vi "stage-controller.vi"() -> ()   [LabVIEW 2014]
uses:
  Stage SubVIs/ctts/move stage.ctl
  stage-controller-globals.vi
  Library Files - Andor and MadCity/Madlib/Madlib.lvlib
panel:
  in  "Current Z 2":ext(slide)=5.551115123125783e-17 scale=-1.0..1.0 scale format="%_1f"
  out "Current (X,Y)":cluster{ext[], ext[]}[](graph)=[{[101.064], [100.915]}, {[101.064, 151.59599999999998], [100.915, 100.915]}, {[101.064, 151.59599999999998], [50.457499999999996, 50.457499999999996]}]
  in  "Field Number":u32(slide)=1 min=1 max=16 step=1 scale=1.0..16.0
  in  "Field Size":enum16{"0", "1", "4", "9", "16"}(ring)=enum."16"
  in  "x-":bool
  in  "y+":bool
  in  "y-":bool
  in  "x+":bool
  out "Current Z (um)":ext=101.117
  out "Current X (um)":ext=101.064
  out "Current Y (um)":ext=100.915
  in  "Current Z":dbl(slide)=101.5 min=0.0 step=0.5 scale=0.0..202.234 scale format="%#_4g"
  out "At limit 3":bool
  out "At limit 2":bool
  out "At limit":bool
  in  "x,y step (um)":ext=10.0 format="%_5g"
  in  "z step (um)":ext(slide)=0.1 scale=0.05..2.0 scale format="%#_2g"
  in  "z-":bool
  in  "z+":bool
  in  "Reset stage to center\n         (x, y, and z)":bool
  in  "STOP":bool
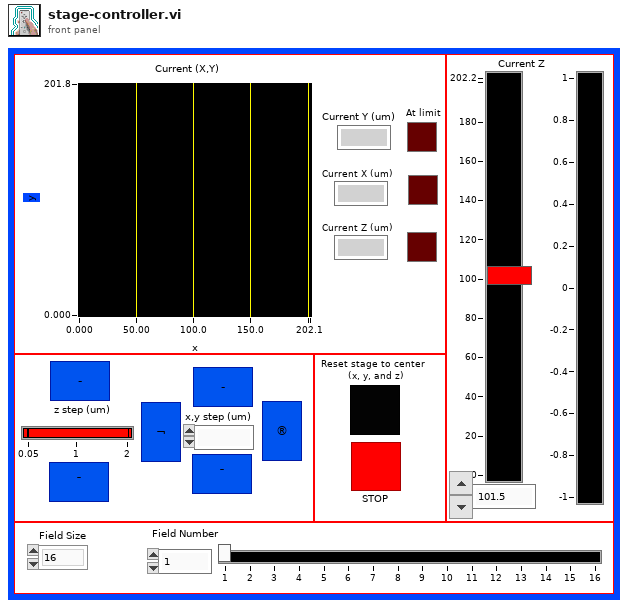
[diagram p1: front panel]
types:
  T1 = cluster{"X Command":dbl, "Y Command":dbl, "Z Command":dbl, "X Position":dbl, "Y Position":dbl, "Z Position":dbl, "X Calibration":dbl, "Y Calibration":dbl, "Z Calibration":dbl}
  T2 = typedef "move stage.ctl" = cluster{"dx (um) (0 -> ignore)":ext, "dy (um) (0 -> ignore)":ext, "dz (um) (0 -> ignore)":ext, "Re-center x,y":bool, "Re-center z":bool, "x (um) (-1 -> ignore)":dbl, "y (um) (-1 -> ignore)":dbl, "z (um) (-1 -> ignore)":dbl, "Move to Next Field":bool}
  T3 = typedef "small z increment.ctl" = dbl
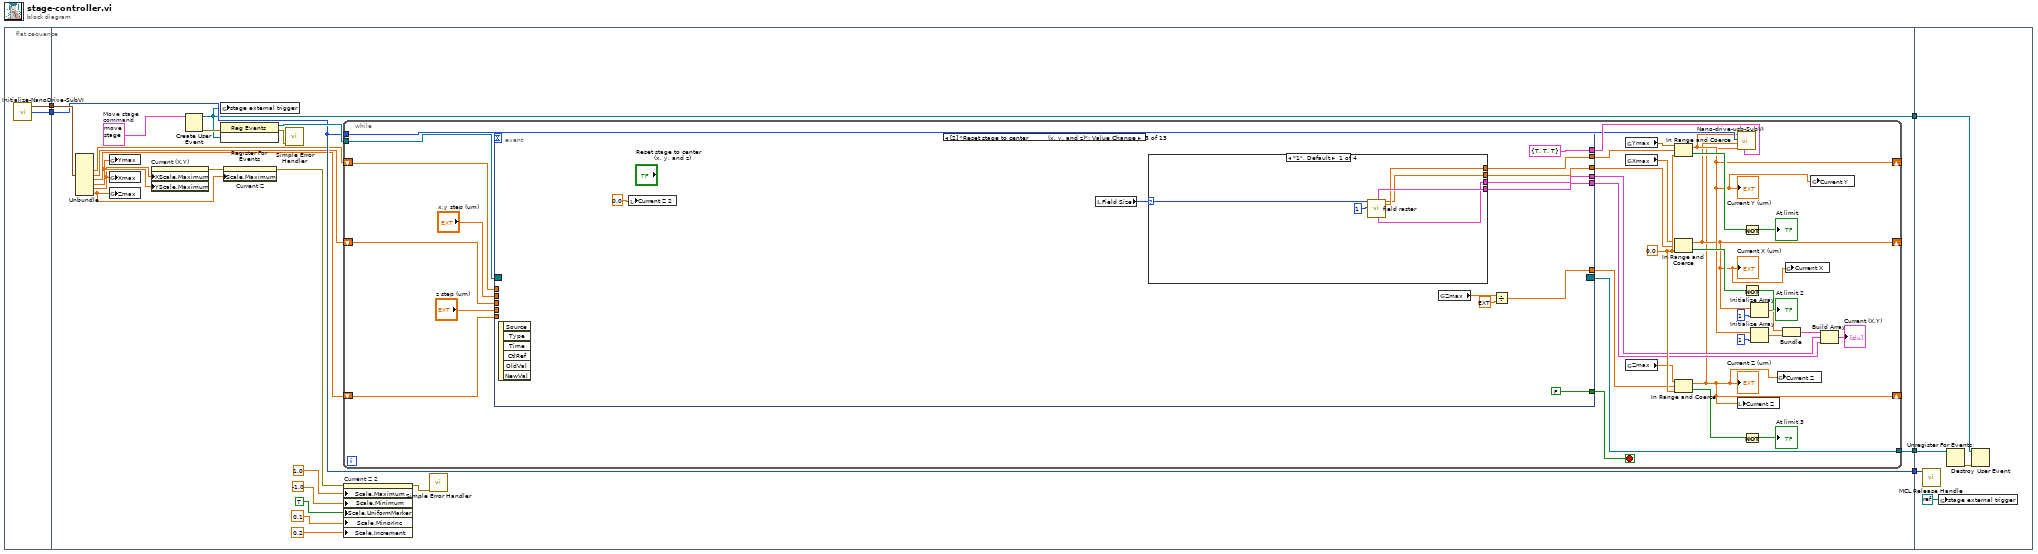
[diagram p0: block diagram]
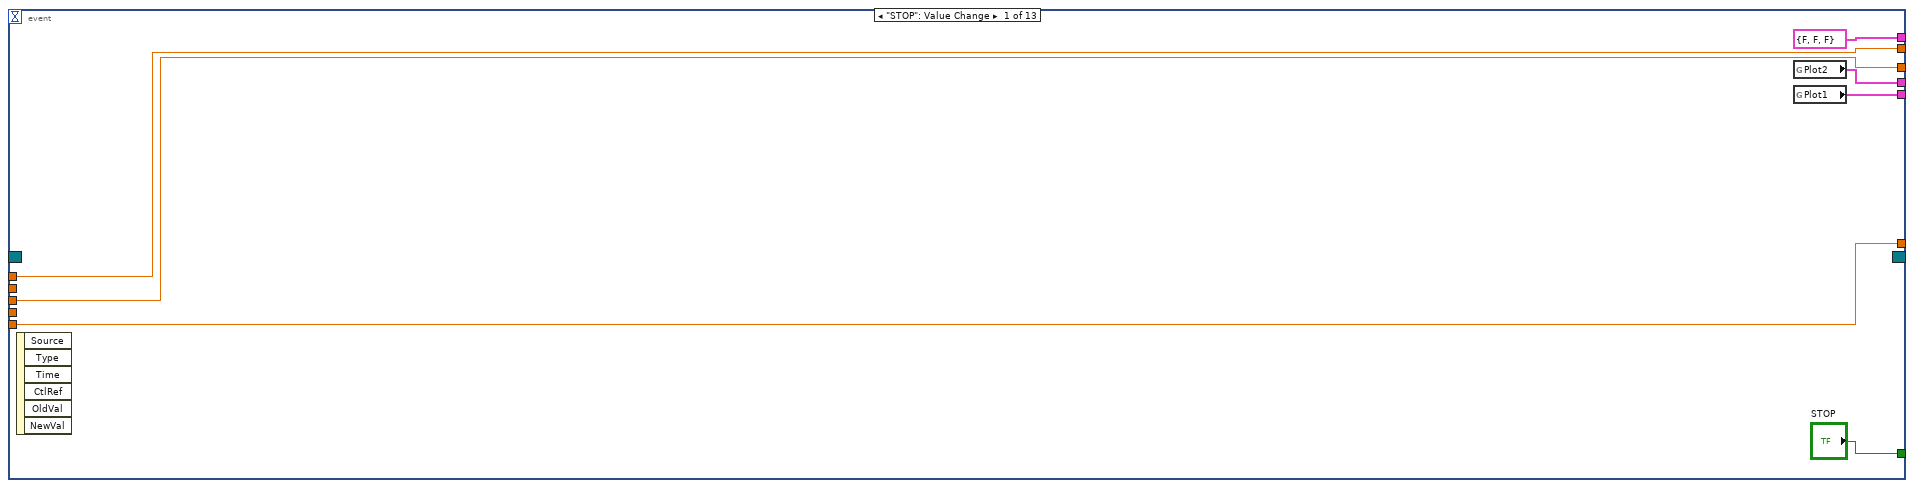
[diagram p2: hidden frame]
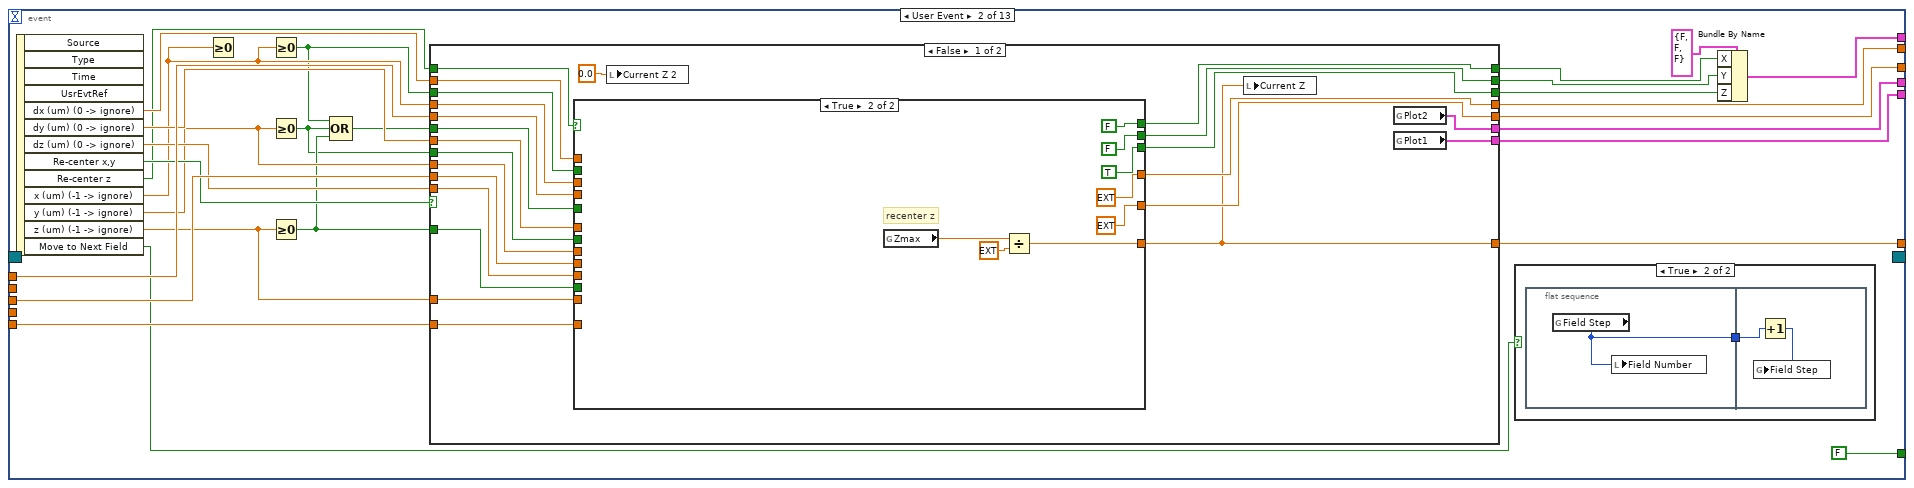
[diagram p3: hidden frame]
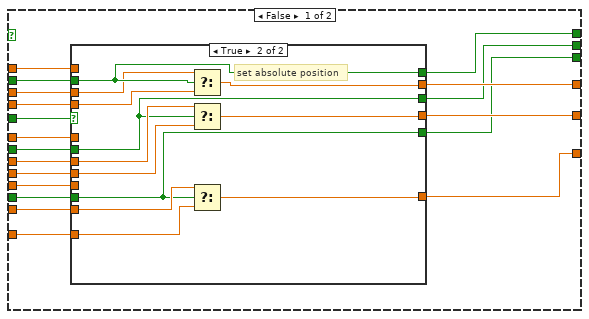
[diagram p5: hidden frame]
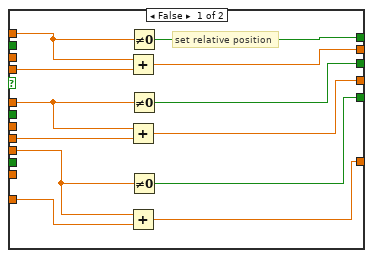
[diagram p6: hidden frame]
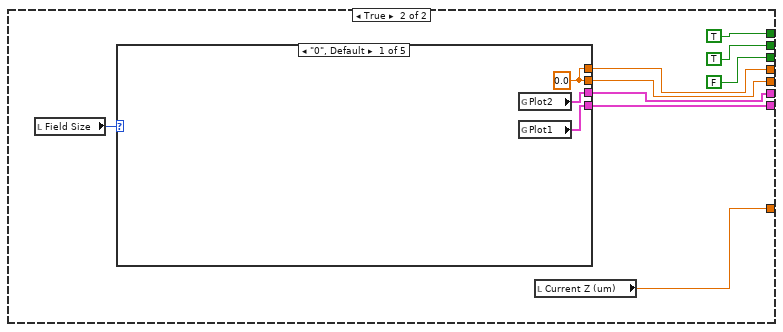
[diagram p7: hidden frame]
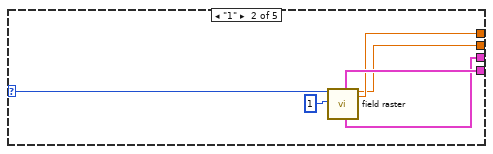
[diagram p8: hidden frame]
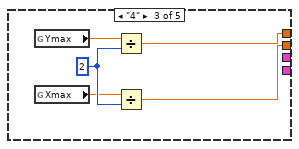
[diagram p9: hidden frame]
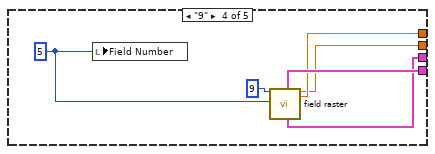
[diagram p10: hidden frame]
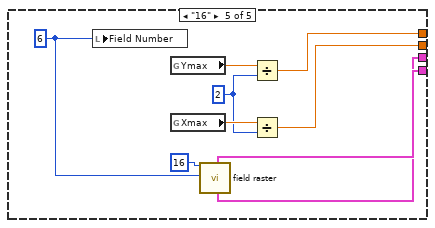
[diagram p11: hidden frame]
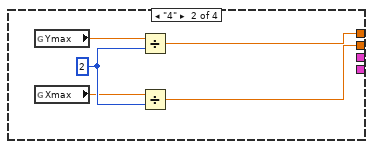
[diagram p12: hidden frame]
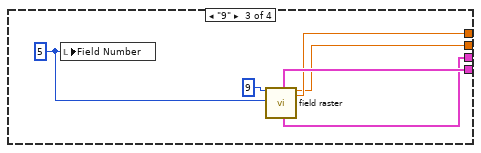
[diagram p13: hidden frame]
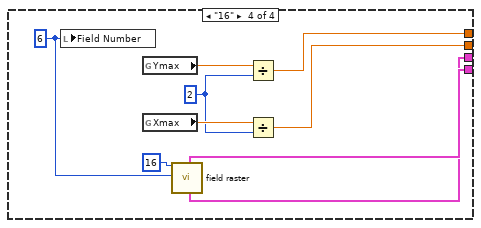
[diagram p14: hidden frame]
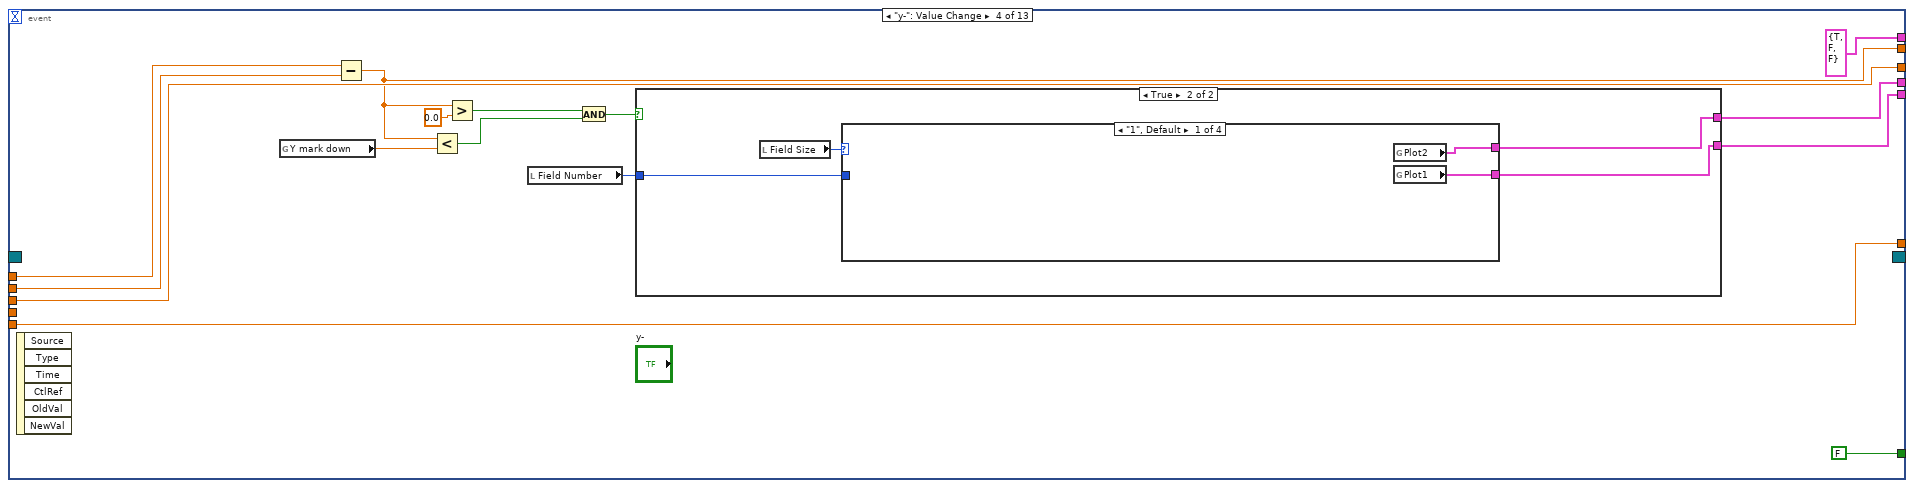
[diagram p15: hidden frame]
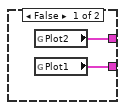
[diagram p16: hidden frame]
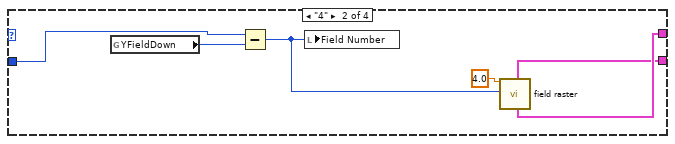
[diagram p17: hidden frame]
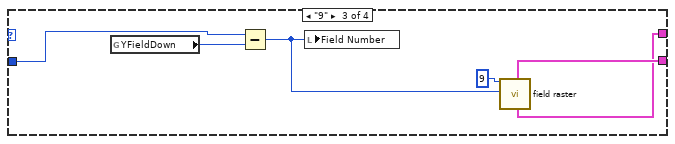
[diagram p18: hidden frame]
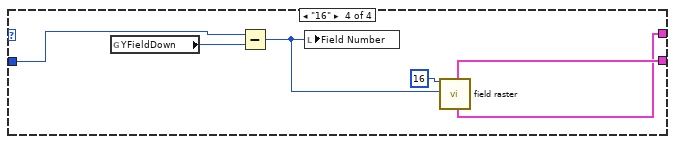
[diagram p19: hidden frame]
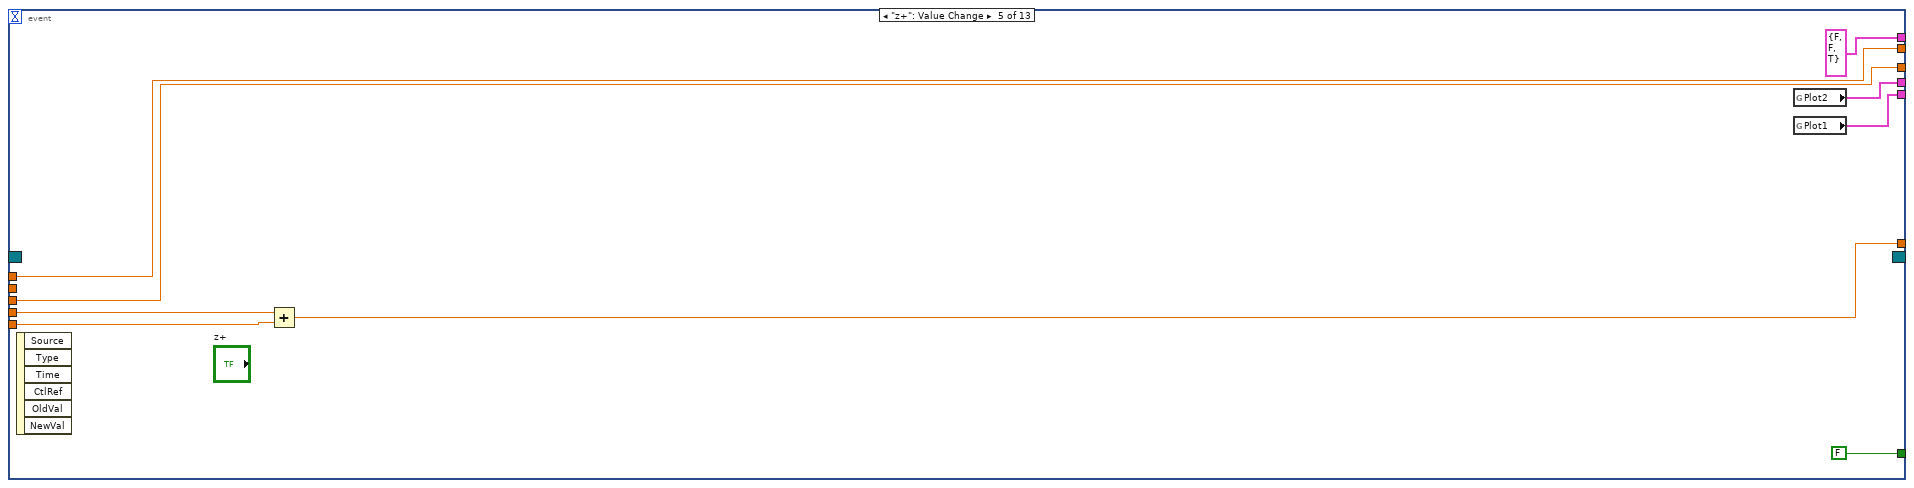
[diagram p20: hidden frame]
diagram:
  n1 = flat-sequence {
    tunnel: [w7] -> w5
    tunnel: [w6] -> w2
    tunnel: w5 -> [w29]
    tunnel: [w24] -> w4
    tunnel: [w8] -> w3
    tunnel: w2 -> [w23]
    tunnel: [w23] -> w1
    tunnel: w4 -> [w498]
    tunnel: w3 -> [w497]
    tunnel: w1 -> [w496]
    frame #0 {
      n2 = call "Initialize-NanoDrive-SubVI.vi"() -> ("Output Pos Info"=w7:T1, "Handle"=w6:i32)  [unwired: 1 in, 1 out]
    }
    frame #1 {
      w28 = T2 {"dx (um) (0 -> ignore)"=0.0, "dy (um) (0 -> ignore)"=0.0, "dz (um) (0 -> ignore)"=0.0, "Re-center x,y"=FALSE, "Re-center z"=FALSE, "x (um) (-1 -> ignore)"=-1.0, "y (um) (-1 -> ignore)"=-1.0, "z (um) (-1 -> ignore)"=-1.0, "Move to Next Field"=FALSE}  # Move stage command
      n3 = Unbundle(w29) -> ("X Position"=w22:dbl, "Y Position"=w21:dbl, "Z Position"=w20:dbl, "X Calibration"=w18:dbl, "Y Calibration"=w17:dbl, "Z Calibration"=w16:dbl)  [unwired: 3 out]
      n4 = global write "stage-controller-globals.vi" "Ymax"(w18) -> ()
      n5 = global write "stage-controller-globals.vi" "Xmax"(w17) -> ()
      n6 = global write "stage-controller-globals.vi" "Zmax"(w16) -> ()
      n7 = property on="Current (X,Y)" class="XYGraph (strict)"("XScale.Maximum"=w17, "YScale.Maximum"=w18) -> (error out=w19:errorcluster)  [unwired: 2 in, 1 out]
      n8 = Create User Event(user event datatype=w28) -> (user event=w8:refnum<user-event>, error out=w26:errorcluster)  [unwired: 1 in]
      n9 = global write "stage-controller-globals.vi" "stage external trigger"(w8) -> ()
      n10 = register-events(error in=w26, w8) -> (reference out=w25:refnum<event-registration>, error out=w27:errorcluster)  [unwired: 1 in]
      n11 = property on="Current Z" class="Slide (strict)"(error in=w19, "Scale.Maximum"=w16) -> (error out=w15:errorcluster)  [unwired: 1 in, 1 out]
      n12 = call <vilib>:"Simple Error Handler.vi"("error in (no error)"=w27) -> ()  [unwired: 1 in, 8 out]
      n13 = while {
        tunnel: w25 -> [w61]
        tunnel: [w60] -> w24
        tunnel: w23 -> [w46]
        shift-right: [w32] -> _
        shift-left: w22 -> [w45]
        shift-right: [w31] -> _
        shift-left: w21 -> [w44]
        shift-right: [w30] -> _
        shift-left: w20 -> [w43]
        stop <- w62 stop-if-true
        w59 = 0.0
        n14 = event shown="[2] \"Reset stage to center          (x, y, and z)\": Value Change" {
          selector: w61 -> [_ _ _ _ _ _ _ _ _ _ _ _ _]
          dyn-events: [_ _ _ _ _ _ _ _ _ _ _ _ _] -> w60
          timeout: _ -> [_ _ _ _ _ _ _ _ _ _ _ _ _]
          tunnel: ["STOP" FALSE ("Stop") FALSE ("Stop") FALSE ("Stop") FALSE ("Stop") FALSE ("Stop") FALSE ("Stop") FALSE ("Stop") FALSE ("Stop") FALSE ("Stop") FALSE ("Stop") FALSE FALSE] -> w62
          tunnel: w45 -> [w69 w97 _ w261 w299 w306 w317 w336 w347 w392 w430 _ _]
          tunnel: w44 -> [w68 w96 _ w264 w294 w305 w316 w335 w351 w389 w434 _ _]
          tunnel: w43 -> [w67 w95 _ w263 w296 _ w314 w332 w352 w393 w433 _ _]
          tunnel: [w69 w92 w216 w252 w299 w306 w317 w336 w347 w392 w422 w465 w488] -> w58
          tunnel: [w68 w93 w217 w264 w294 w305 w316 w335 w340 w381 w434 w464 w487] -> w57
          tunnel: [w67 w94 w222 w263 w298 "Current Z" w313 w338 w352 w393 w433 w468 w483] -> w56
          tunnel: [cluster{"X":bool, "Y":bool, "Z":bool} {"X"=FALSE, "Y"=FALSE, "Z"=FALSE} ("Set this axis?") w85 cluster{"X":bool, "Y":bool, "Z":bool} {"X"=TRUE, "Y"=TRUE, "Z"=TRUE} ("Set this axis?") cluster{"X":bool, "Y":bool, "Z":bool} {"X"=TRUE, "Y"=FALSE, "Z"=FALSE} ("Set this axis?") cluster{"X":bool, "Y":bool, "Z":bool} {"X"=FALSE, "Y"=FALSE, "Z"=TRUE} ("Set this axis?") cluster{"X":bool, "Y":bool, "Z":bool} {"X"=FALSE, "Y"=FALSE, "Z"=TRUE} ("Set this axis?") cluster{"X":bool, "Y":bool, "Z":bool} {"X"=FALSE, "Y"=FALSE, "Z"=TRUE} ("Set this axis?") cluster{"X":bool, "Y":bool, "Z":bool} {"X"=FALSE, "Y"=FALSE, "Z"=TRUE} ("Set this axis?") cluster{"X":bool, "Y":bool, "Z":bool} {"X"=FALSE, "Y"=TRUE, "Z"=FALSE} ("Set this axis?") cluster{"X":bool, "Y":bool, "Z":bool} {"X"=FALSE, "Y"=TRUE, "Z"=FALSE} ("Set this axis?") cluster{"X":bool, "Y":bool, "Z":bool} {"X"=TRUE, "Y"=FALSE, "Z"=FALSE} ("Set this axis?") cluster{"X":bool, "Y":bool, "Z":bool} {"X"=FALSE, "Y"=FALSE, "Z"=FALSE} ("Set this axis?") cluster{"X":bool, "Y":bool, "Z":bool} {"X"=TRUE, "Y"=TRUE, "Z"=FALSE} ("Set this axis?")] -> w47
          tunnel: "x,y step (um)" -> [_ _ _ w260 _ _ _ _ w350 w390 w431 _ _]
          tunnel: "z step (um)" -> [_ _ _ _ w295 _ _ w333 _ _ _ _ _]
          tunnel: [w64 w72 w219 w257 w293 w302 w320 w331 w345 w386 w427 w463 w489] -> w38
          tunnel: [w65 w73 w220 w258 w292 w303 w319 w330 w346 w387 w428 w462 w490] -> w37
          event "STOP": Value Change {
            n15 = event-data() -> ()  [unwired: 7 out]
            n16 = global read "stage-controller-globals.vi" "Plot2"() -> (w64:cluster{dbl[], dbl[]})
            n17 = global read "stage-controller-globals.vi" "Plot1"() -> (w65:cluster{dbl[], dbl[]})
          }
          event User Event {
            n18 = event-data() -> ("dx (um) (0 -> ignore)"=w90:ext, "dy (um) (0 -> ignore)"=w89:ext, "dz (um) (0 -> ignore)"=w88:ext, "Re-center x,y"=w87:bool, "Re-center z"=w81:bool, "x (um) (-1 -> ignore)"=w77:dbl, "y (um) (-1 -> ignore)"=w78:dbl, "z (um) (-1 -> ignore)"=w79:dbl, "Move to Next Field"=w71:bool)  [unwired: 5 out]
            n19 = Greater Or Equal To 0?(x=w77) -> ()  [unwired: 1 out]
            n20 = Greater Or Equal To 0?(x=w77) -> (x >= 0?=w74:bool)
            n21 = Greater Or Equal To 0?(x=w78) -> (x >= 0?=w75:bool)
            n22 = Greater Or Equal To 0?(x=w79) -> (x >= 0?=w76:bool)
            n23 = Compound Arithmetic op=OR(w74, w75, w76) -> (w80:bool)
            n24 = case shown="False" w87 {
              tunnel: w97 -> [w124 _]
              tunnel: w96 -> [w123 _]
              tunnel: w95 -> [w122 _]
              tunnel: [w105 w177] -> w94
              tunnel: [w121 w179] -> w93
              tunnel: [w120 w178] -> w92
              tunnel: w90 -> [w119 _]
              tunnel: w89 -> [w118 _]
              tunnel: w88 -> [w117 _]
              tunnel: [w116 FALSE] -> w84
              tunnel: [w115 TRUE] -> w83
              tunnel: [w114 TRUE] -> w82
              tunnel: w81 -> [w113 _]
              tunnel: w80 -> [w112 _]
              tunnel: w79 -> [w111 _]
              tunnel: w78 -> [w110 _]
              tunnel: w77 -> [w109 _]
              tunnel: w76 -> [w108 _]
              tunnel: w75 -> [w107 _]
              tunnel: w74 -> [w106 _]
              tunnel: [w103 w181] -> w73
              tunnel: [w102 w180] -> w72
              frame False {
                n25 = case shown="True" w113 {
                  tunnel: w124 -> [w143 _]
                  tunnel: w123 -> [w142 _]
                  tunnel: w122 -> [w141 _]
                  tunnel: [w140 w174] -> w105
                  tunnel: [w139 ext 0.0] -> w121
                  tunnel: [w138 ext 0.0] -> w120
                  tunnel: w119 -> [w137 _]
                  tunnel: w118 -> [w136 _]
                  tunnel: w117 -> [w135 _]
                  tunnel: [w134 TRUE] -> w116
                  tunnel: [w133 FALSE] -> w115
                  tunnel: [w132 FALSE] -> w114
                  tunnel: w112 -> [w131 _]
                  tunnel: w111 -> [w130 _]
                  tunnel: w110 -> [w129 _]
                  tunnel: w109 -> [w128 _]
                  tunnel: w108 -> [w127 _]
                  tunnel: w107 -> [w126 _]
                  tunnel: w106 -> [w125 _]
                  frame False {
                    n26 = case shown="True" w131 {
                      tunnel: w143 -> [w155 w163]
                      tunnel: w142 -> [w154 w160]
                      tunnel: w141 -> [w153 w157]
                      tunnel: [w152 w159] -> w140
                      tunnel: [w151 w162] -> w139
                      tunnel: [w150 w166] -> w138
                      tunnel: w137 -> [w149 _]
                      tunnel: w136 -> [w148 _]
                      tunnel: w135 -> [w147 _]
                      tunnel: [w146 w156] -> w134
                      tunnel: [w145 w161] -> w133
                      tunnel: [w144 w165] -> w132
                      tunnel: w130 -> [_ w158]
                      tunnel: w129 -> [_ w167]
                      tunnel: w128 -> [_ w164]
                      tunnel: w127 -> [_ w156]
                      tunnel: w126 -> [_ w161]
                      tunnel: w125 -> [_ w165]
                      frame False {
                        # "set relative position"
                        n27 = Add(x=w149, y=w155) -> (x+y=w150:ext)
                        n28 = Add(x=w148, y=w154) -> (x+y=w151:ext)
                        n29 = Add(x=w147, y=w153) -> (x+y=w152:ext)
                        n30 = Not Equal To 0?(x=w149) -> (x != 0?=w144:bool)
                        n31 = Not Equal To 0?(x=w148) -> (x != 0?=w145:bool)
                        n32 = Not Equal To 0?(x=w147) -> (x != 0?=w146:bool)
                      }
                      frame True {
                        # "set absolute position"
                        n33 = Select(t=w164, s=w165, f=w163) -> (s? t:f=w166:ext)
                        n34 = Select(t=w167, s=w161, f=w160) -> (s? t:f=w162:ext)
                        n35 = Select(t=w158, s=w156, f=w157) -> (s? t:f=w159:ext)
                      }
                    }
                  }
                  frame True {
                    # "recenter z"
                    n36 = global read "stage-controller-globals.vi" "Zmax"() -> (w168:dbl)
                    n37 = Divide(x=w168, y=ext 2.0) -> (x/y=w174:ext)
                  }
                }
                n38 = local write "Current Z 2"(0.0) -> ()
                n39 = local write "Current Z"(w105) -> ()
                n40 = global read "stage-controller-globals.vi" "Plot2"() -> (w102:cluster{dbl[], dbl[]})
                n41 = global read "stage-controller-globals.vi" "Plot1"() -> (w103:cluster{dbl[], dbl[]})
              }
              frame True {
                n42 = local read "Field Size"() -> (w176:enum16{"0", "1", "4", "9", "16"})
                n43 = case shown="\"0\", Default" w176 {
                  selector: w176 -> [_ w191 _ _ _]
                  tunnel: [w186 w193 _ w202 w208] -> w181
                  tunnel: [w187 w192 _ w201 w207] -> w180
                  tunnel: [w185 w189 w198 w200 w211] -> w178
                  tunnel: [w185 w188 w197 w199 w210] -> w179
                  frame "0", Default {
                    w185 = 0.0
                    n44 = global read "stage-controller-globals.vi" "Plot2"() -> (w187:cluster{dbl[], dbl[]})
                    n45 = global read "stage-controller-globals.vi" "Plot1"() -> (w186:cluster{dbl[], dbl[]})
                  }
                  frame "1" {
                    n46 = call "field raster.vi"("field size"=w191, "field number"=1) -> ("Plot1"=w193:cluster{dbl[], dbl[]}, "Plot2"=w192:cluster{dbl[], dbl[]}, "current Y"=w188:dbl, "current X"=w189:dbl)  [unwired: 12 in, 2 out]
                  }
                  frame "4" {
                    w196 = 2
                    n47 = global read "stage-controller-globals.vi" "Ymax"() -> (w194:dbl)
                    n48 = global read "stage-controller-globals.vi" "Xmax"() -> (w195:dbl)
                    n49 = Divide(x=w194, y=w196) -> (x/y=w198:dbl)
                    n50 = Divide(x=w195, y=w196) -> (x/y=w197:dbl)
                  }
                  frame "9" {
                    w203 = 5
                    n51 = local write "Field Number"(w203) -> ()
                    n52 = call "field raster.vi"("field size"=9, "field number"=w203) -> ("Plot1"=w202:cluster{dbl[], dbl[]}, "Plot2"=w201:cluster{dbl[], dbl[]}, "current Y"=w199:dbl, "current X"=w200:dbl)  [unwired: 12 in, 2 out]
                  }
                  frame "16" {
                    w206 = 2
                    w205 = 6
                    n53 = local write "Field Number"(w205) -> ()
                    n54 = global read "stage-controller-globals.vi" "Ymax"() -> (w213:dbl)
                    n55 = global read "stage-controller-globals.vi" "Xmax"() -> (w212:dbl)
                    n56 = call "field raster.vi"("field size"=16, "field number"=w205) -> ("Plot1"=w208:cluster{dbl[], dbl[]}, "Plot2"=w207:cluster{dbl[], dbl[]})  [unwired: 12 in, 4 out]
                    n57 = Divide(x=w213, y=w206) -> (x/y=w211:dbl)
                    n58 = Divide(x=w212, y=w206) -> (x/y=w210:dbl)
                  }
                }
                n59 = local read "Current Z (um)"() -> (w177:ext)
              }
            }
            n60 = case shown="True" w71 {
              frame False {
              }
              frame True {
                n61 = flat-sequence {
                  tunnel: [w99] -> w98
                  tunnel: w98 -> [w101]
                  frame #0 {
                    n62 = global read "stage-controller-globals.vi" "Field Step"() -> (w99:u32)
                    n63 = local write "Field Number"(w99) -> ()
                  }
                  frame #1 {
                    n64 = Increment(x=w101) -> (x+1=w100:u32)
                    n65 = global write "stage-controller-globals.vi" "Field Step"(w100) -> ()
                  }
                }
              }
            }
            n66 = Bundle By Name(cluster=cluster{"X":bool, "Y":bool, "Z":bool} {"X"=FALSE, "Y"=FALSE, "Z"=FALSE} ("Set this axis?"), "X"=w82, "Y"=w83, "Z"=w84) -> (w85:cluster{"X":bool, "Y":bool, "Z":bool})
          }
          event "Reset stage to center\n         (x, y, and z)": Value Change {
            n67 = event-data() -> ()  [unwired: 7 out]
            n68 = local write "Current Z 2"(0.0) -> ()
            n69 = local read "Field Size"() -> (w218:enum16{"0", "1", "4", "9", "16"})
            n70 = case shown="\"1\", Default" w218 {
              selector: w218 -> [w228 _ _ _]
              tunnel: [w230 _ w239 w245] -> w220
              tunnel: [w229 _ w238 w244] -> w219
              tunnel: [w226 w235 w237 w248] -> w216
              tunnel: [w225 w234 w236 w247] -> w217
              frame "1", Default {
                n71 = call "field raster.vi"("field size"=w228, "field number"=1) -> ("Plot1"=w230:cluster{dbl[], dbl[]}, "Plot2"=w229:cluster{dbl[], dbl[]}, "current Y"=w225:dbl, "current X"=w226:dbl)  [unwired: 12 in, 2 out]
              }
              frame "4" {
                w233 = 2
                n72 = global read "stage-controller-globals.vi" "Ymax"() -> (w231:dbl)
                n73 = global read "stage-controller-globals.vi" "Xmax"() -> (w232:dbl)
                n74 = Divide(x=w231, y=w233) -> (x/y=w235:dbl)
                n75 = Divide(x=w232, y=w233) -> (x/y=w234:dbl)
              }
              frame "9" {
                w240 = 5
                n76 = local write "Field Number"(w240) -> ()
                n77 = call "field raster.vi"("field size"=9, "field number"=w240) -> ("Plot1"=w239:cluster{dbl[], dbl[]}, "Plot2"=w238:cluster{dbl[], dbl[]}, "current Y"=w236:dbl, "current X"=w237:dbl)  [unwired: 12 in, 2 out]
              }
              frame "16" {
                w243 = 2
                w242 = 6
                n78 = local write "Field Number"(w242) -> ()
                n79 = global read "stage-controller-globals.vi" "Ymax"() -> (w250:dbl)
                n80 = global read "stage-controller-globals.vi" "Xmax"() -> (w249:dbl)
                n81 = call "field raster.vi"("field size"=16, "field number"=w242) -> ("Plot1"=w245:cluster{dbl[], dbl[]}, "Plot2"=w244:cluster{dbl[], dbl[]})  [unwired: 12 in, 4 out]
                n82 = Divide(x=w250, y=w243) -> (x/y=w248:dbl)
                n83 = Divide(x=w249, y=w243) -> (x/y=w247:dbl)
              }
            }
            n84 = global read "stage-controller-globals.vi" "Zmax"() -> (w215:dbl)
            n85 = Divide(x=w215, y=ext 2.0) -> (x/y=w222:ext)
          }
          event "y-": Value Change {
            n86 = event-data() -> ()  [unwired: 7 out]
            n87 = global read "stage-controller-globals.vi" "Y mark down"() -> (w259:dbl)
            n88 = Subtract(x=w261, y=w260) -> (x-y=w252:ext)
            n89 = Less?(x=w252, y=w259) -> (x < y?=w256:bool)
            n90 = Greater?(x=w252, y=0.0) -> (0:w254:bool)
            n91 = local read "Field Number"() -> (w251:u32)
            n92 = And(x=w254, y=w256) -> (x .and. y?=w255:bool)
            n93 = case shown="True" w255 {
              tunnel: [w267 w270] -> w258
              tunnel: [w266 w269] -> w257
              tunnel: w251 -> [_ w268]
              frame False {
                n94 = global read "stage-controller-globals.vi" "Plot2"() -> (w266:cluster{dbl[], dbl[]})
                n95 = global read "stage-controller-globals.vi" "Plot1"() -> (w267:cluster{dbl[], dbl[]})
              }
              frame True {
                n96 = local read "Field Size"() -> (w271:enum16{"0", "1", "4", "9", "16"})
                n97 = case shown="\"1\", Default" w271 {
                  tunnel: w268 -> [_ w275 w285 w290]
                  tunnel: [w273 w278 w283 w288] -> w270
                  tunnel: [w272 w279 w282 w287] -> w269
                  frame "1", Default {
                    n98 = global read "stage-controller-globals.vi" "Plot2"() -> (w272:cluster{dbl[], dbl[]})
                    n99 = global read "stage-controller-globals.vi" "Plot1"() -> (w273:cluster{dbl[], dbl[]})
                  }
                  frame "4" {
                    n100 = global read "stage-controller-globals.vi" "YFieldDown"() -> (w274:u32)
                    n101 = Subtract(x=w275, y=w274) -> (x-y=w276:u32)
                    n102 = local write "Field Number"(w276) -> ()
                    n103 = call "field raster.vi"("field size"=4.0, "field number"=w276) -> ("Plot1"=w278:cluster{dbl[], dbl[]}, "Plot2"=w279:cluster{dbl[], dbl[]})  [unwired: 12 in, 4 out]
                  }
                  frame "9" {
                    n104 = global read "stage-controller-globals.vi" "YFieldDown"() -> (w281:u32)
                    n105 = Subtract(x=w285, y=w281) -> (x-y=w280:u32)
                    n106 = local write "Field Number"(w280) -> ()
                    n107 = call "field raster.vi"("field size"=9, "field number"=w280) -> ("Plot1"=w283:cluster{dbl[], dbl[]}, "Plot2"=w282:cluster{dbl[], dbl[]})  [unwired: 12 in, 4 out]
                  }
                  frame "16" {
                    n108 = global read "stage-controller-globals.vi" "YFieldDown"() -> (w286:u32)
                    n109 = Subtract(x=w290, y=w286) -> (x-y=w289:u32)
                    n110 = local write "Field Number"(w289) -> ()
                    n111 = call "field raster.vi"("field size"=16, "field number"=w289) -> ("Plot1"=w288:cluster{dbl[], dbl[]}, "Plot2"=w287:cluster{dbl[], dbl[]})  [unwired: 12 in, 4 out]
                  }
                }
              }
            }
          }
          event "z+": Value Change {
            n112 = event-data() -> ()  [unwired: 7 out]
            n113 = Add(x=w295, y=w296) -> (x+y=w298:ext)
            n114 = global read "stage-controller-globals.vi" "Plot2"() -> (w293:cluster{dbl[], dbl[]})
            n115 = global read "stage-controller-globals.vi" "Plot1"() -> (w292:cluster{dbl[], dbl[]})
          }
          event "Current Z": Mouse Up {
            w301 = 0.0
            n116 = event-data() -> ()  [unwired: 5 out]
            n117 = global write "stage-controller-globals.vi" "Previous\nsmall Z increment"(w301) -> ()
            n118 = local write "Current Z 2"(w301) -> ()
            n119 = global read "stage-controller-globals.vi" "Plot2"() -> (w302:cluster{dbl[], dbl[]})
            n120 = global read "stage-controller-globals.vi" "Plot1"() -> (w303:cluster{dbl[], dbl[]})
          }
          event "Current Z 2": Mouse Up {
            n121 = event-data() -> ()  [unwired: 8 out]
            n122 = global read "stage-controller-globals.vi" "Previous\nsmall Z increment"() -> (w312:T3)
            n123 = Subtract(x="Current Z 2", y=w312) -> (x-y=w310:ext)
            n124 = Greater?(x=w310, y=0.0) -> (0:w315:bool)
            n125 = case shown="False" w315 {
              tunnel: w314 -> [w322 w328]
              tunnel: w310 -> [w323 w327]
              tunnel: [w325 w329] -> w313
              tunnel: "Current Z 2" -> [w324 w326]
              frame False {
                n126 = global write "stage-controller-globals.vi" "Previous\nsmall Z increment"(w324) -> ()
                n127 = Add(x=w322, y=w323) -> (x+y=w325:ext)
              }
              frame True {
                n128 = global write "stage-controller-globals.vi" "Previous\nsmall Z increment"(w326) -> ()
                n129 = Add(x=w328, y=w327) -> (x+y=w329:ext)
              }
            }
            n130 = global read "stage-controller-globals.vi" "Plot2"() -> (w320:cluster{dbl[], dbl[]})
            n131 = global read "stage-controller-globals.vi" "Plot1"() -> (w319:cluster{dbl[], dbl[]})
          }
          event "z-": Value Change {
            n132 = event-data() -> ()  [unwired: 7 out]
            n133 = Subtract(x=w332, y=w333) -> (x-y=w338:ext)
            n134 = global read "stage-controller-globals.vi" "Plot2"() -> (w331:cluster{dbl[], dbl[]})
            n135 = global read "stage-controller-globals.vi" "Plot1"() -> (w330:cluster{dbl[], dbl[]})
          }
          event "x+": Value Change {
            n136 = event-data() -> ()  [unwired: 7 out]
            n137 = Add(x=w350, y=w351) -> (x+y=w340:ext)
            n138 = global read "stage-controller-globals.vi" "X mark up"() -> (w348:dbl)
            n139 = global read "stage-controller-globals.vi" "Xmax"() -> (w341:dbl)
            n140 = Less?(x=w340, y=w341) -> (x < y?=w342:bool)
            n141 = Greater?(x=w340, y=w348) -> (0:w343:bool)
            n142 = local read "Field Number"() -> (w339:u32)
            n143 = And(x=w342, y=w343) -> (x .and. y?=w344:bool)
            n144 = case shown="True" w344 {
              tunnel: [w355 w358] -> w346
              tunnel: [w354 w357] -> w345
              tunnel: w339 -> [_ w356]
              frame False {
                n145 = global read "stage-controller-globals.vi" "Plot2"() -> (w354:cluster{dbl[], dbl[]})
                n146 = global read "stage-controller-globals.vi" "Plot1"() -> (w355:cluster{dbl[], dbl[]})
              }
              frame True {
                n147 = local read "Field Size"() -> (w359:enum16{"0", "1", "4", "9", "16"})
                n148 = case shown="\"1\", Default" w359 {
                  tunnel: w356 -> [_ w363 w373 w378]
                  tunnel: [w361 w366 w371 w376] -> w358
                  tunnel: [w360 w367 w370 w375] -> w357
                  frame "1", Default {
                    n149 = global read "stage-controller-globals.vi" "Plot1"() -> (w360:cluster{dbl[], dbl[]})
                    n150 = global read "stage-controller-globals.vi" "Plot1"() -> (w361:cluster{dbl[], dbl[]})
                  }
                  frame "4" {
                    n151 = global read "stage-controller-globals.vi" "XFieldDiff"() -> (w362:dbl)
                    n152 = Add(x=w363, y=w362) -> (x+y=w364:dbl)
                    n153 = local write "Field Number"(w364) -> ()
                    n154 = call "field raster.vi"("field size"=4.0, "field number"=w364) -> ("Plot1"=w366:cluster{dbl[], dbl[]}, "Plot2"=w367:cluster{dbl[], dbl[]})  [unwired: 12 in, 4 out]
                  }
                  frame "9" {
                    n155 = global read "stage-controller-globals.vi" "XFieldDiff"() -> (w368:dbl)
                    n156 = Add(x=w373, y=w368) -> (x+y=w369:dbl)
                    n157 = local write "Field Number"(w369) -> ()
                    n158 = call "field raster.vi"("field size"=9, "field number"=w369) -> ("Plot1"=w371:cluster{dbl[], dbl[]}, "Plot2"=w370:cluster{dbl[], dbl[]})  [unwired: 12 in, 4 out]
                  }
                  frame "16" {
                    n159 = global read "stage-controller-globals.vi" "XFieldDiff"() -> (w374:dbl)
                    n160 = Add(x=w378, y=w374) -> (x+y=w377:dbl)
                    n161 = local write "Field Number"(w377) -> ()
                    n162 = call "field raster.vi"("field size"=16, "field number"=w377) -> ("Plot1"=w376:cluster{dbl[], dbl[]}, "Plot2"=w375:cluster{dbl[], dbl[]})  [unwired: 12 in, 4 out]
                  }
                }
              }
            }
          }
          event "x-": Value Change {
            n163 = event-data() -> ()  [unwired: 7 out]
            n164 = global read "stage-controller-globals.vi" "X mark down"() -> (w388:dbl)
            n165 = Subtract(x=w389, y=w390) -> (x-y=w381:ext)
            n166 = Less?(x=w381, y=w388) -> (x < y?=w384:bool)
            n167 = Greater?(x=w381, y=ext 0.0) -> (0:w383:bool)
            n168 = local read "Field Number"() -> (w380:u32)
            n169 = And(x=w383, y=w384) -> (x .and. y?=w385:bool)
            n170 = case shown="True" w385 {
              tunnel: [w396 w399] -> w387
              tunnel: [w395 w398] -> w386
              tunnel: w380 -> [_ w397]
              frame False {
                n171 = global read "stage-controller-globals.vi" "Plot2"() -> (w395:cluster{dbl[], dbl[]})
                n172 = global read "stage-controller-globals.vi" "Plot1"() -> (w396:cluster{dbl[], dbl[]})
              }
              frame True {
                n173 = local read "Field Size"() -> (w400:enum16{"0", "1", "4", "9", "16"})
                n174 = case shown="\"1\", Default" w400 {
                  tunnel: w397 -> [_ w404 w414 w419]
                  tunnel: [w402 w407 w412 w417] -> w399
                  tunnel: [w401 w408 w411 w416] -> w398
                  frame "1", Default {
                    n175 = global read "stage-controller-globals.vi" "Plot2"() -> (w401:cluster{dbl[], dbl[]})
                    n176 = global read "stage-controller-globals.vi" "Plot1"() -> (w402:cluster{dbl[], dbl[]})
                  }
                  frame "4" {
                    n177 = global read "stage-controller-globals.vi" "XFieldDiff"() -> (w403:dbl)
                    n178 = Subtract(x=w404, y=w403) -> (x-y=w405:dbl)
                    n179 = local write "Field Number"(w405) -> ()
                    n180 = call "field raster.vi"("field size"=4.0, "field number"=w405) -> ("Plot1"=w407:cluster{dbl[], dbl[]}, "Plot2"=w408:cluster{dbl[], dbl[]})  [unwired: 12 in, 4 out]
                  }
                  frame "9" {
                    n181 = global read "stage-controller-globals.vi" "XFieldDiff"() -> (w409:dbl)
                    n182 = Subtract(x=w414, y=w409) -> (x-y=w410:dbl)
                    n183 = local write "Field Number"(w410) -> ()
                    n184 = call "field raster.vi"("field size"=9, "field number"=w410) -> ("Plot1"=w412:cluster{dbl[], dbl[]}, "Plot2"=w411:cluster{dbl[], dbl[]})  [unwired: 12 in, 4 out]
                  }
                  frame "16" {
                    n185 = global read "stage-controller-globals.vi" "XFieldDiff"() -> (w415:dbl)
                    n186 = Subtract(x=w419, y=w415) -> (x-y=w418:dbl)
                    n187 = local write "Field Number"(w418) -> ()
                    n188 = call "field raster.vi"("field size"=16, "field number"=w418) -> ("Plot1"=w417:cluster{dbl[], dbl[]}, "Plot2"=w416:cluster{dbl[], dbl[]})  [unwired: 12 in, 4 out]
                  }
                }
              }
            }
          }
          event "y+": Value Change {
            n189 = event-data() -> ()  [unwired: 7 out]
            n190 = Add(x=w430, y=w431) -> (x+y=w422:ext)
            n191 = global read "stage-controller-globals.vi" "Y mark up"() -> (w429:dbl)
            n192 = global read "stage-controller-globals.vi" "Ymax"() -> (w423:dbl)
            n193 = Less?(x=w422, y=w423) -> (x < y?=w424:bool)
            n194 = Greater?(x=w422, y=w429) -> (0:w425:bool)
            n195 = local read "Field Number"() -> (w421:u32)
            n196 = And(x=w424, y=w425) -> (x .and. y?=w426:bool)
            n197 = case shown="True" w426 {
              tunnel: [w437 w440] -> w428
              tunnel: [w436 w439] -> w427
              tunnel: w421 -> [_ w438]
              frame False {
                n198 = global read "stage-controller-globals.vi" "Plot2"() -> (w436:cluster{dbl[], dbl[]})
                n199 = global read "stage-controller-globals.vi" "Plot1"() -> (w437:cluster{dbl[], dbl[]})
              }
              frame True {
                n200 = local read "Field Size"() -> (w441:enum16{"0", "1", "4", "9", "16"})
                n201 = case shown="\"1\", Default" w441 {
                  tunnel: w438 -> [_ w445 w455 w460]
                  tunnel: [w443 w448 w453 w458] -> w440
                  tunnel: [w442 w449 w452 w457] -> w439
                  frame "1", Default {
                    n202 = global read "stage-controller-globals.vi" "Plot2"() -> (w442:cluster{dbl[], dbl[]})
                    n203 = global read "stage-controller-globals.vi" "Plot1"() -> (w443:cluster{dbl[], dbl[]})
                  }
                  frame "4" {
                    n204 = global read "stage-controller-globals.vi" "YFieldUp"() -> (w444:u32)
                    n205 = Add(x=w445, y=w444) -> (x+y=w446:u32)
                    n206 = local write "Field Number"(w446) -> ()
                    n207 = call "field raster.vi"("field size"=4.0, "field number"=w446) -> ("Plot1"=w448:cluster{dbl[], dbl[]}, "Plot2"=w449:cluster{dbl[], dbl[]})  [unwired: 12 in, 4 out]
                  }
                  frame "9" {
                    n208 = global read "stage-controller-globals.vi" "YFieldUp"() -> (w450:u32)
                    n209 = Add(x=w455, y=w450) -> (x+y=w451:u32)
                    n210 = local write "Field Number"(w451) -> ()
                    n211 = call "field raster.vi"("field size"=9, "field number"=w451) -> ("Plot1"=w453:cluster{dbl[], dbl[]}, "Plot2"=w452:cluster{dbl[], dbl[]})  [unwired: 12 in, 4 out]
                  }
                  frame "16" {
                    n212 = global read "stage-controller-globals.vi" "YFieldUp"() -> (w456:u32)
                    n213 = Add(x=w460, y=w456) -> (x+y=w459:u32)
                    n214 = local write "Field Number"(w459) -> ()
                    n215 = call "field raster.vi"("field size"=16, "field number"=w459) -> ("Plot1"=w458:cluster{dbl[], dbl[]}, "Plot2"=w457:cluster{dbl[], dbl[]})  [unwired: 12 in, 4 out]
                  }
                }
              }
            }
          }
          event "Field Size": Value Change {
            n216 = event-data() -> ()  [unwired: 7 out]
            n217 = flat-sequence {
              tunnel: [w470] -> w466
              tunnel: [w478] -> w462
              tunnel: [w477] -> w463
              tunnel: w466 -> [w474]
              tunnel: [w476] -> w464
              tunnel: [w475] -> w465
              frame #0 {
                w471 = 1
                n218 = Square(x="Field Size") -> (x^2=w470:u16)
                n219 = global write "stage-controller-globals.vi" "Field Size"("Field Size") -> ()
                n220 = property on="Field Number" class="Slide (strict)"("Maximum"=w470, "Minimum"=w471, "Scale.Minimum"=w471, "Scale.Maximum"=w470) -> ()  [unwired: 2 in, 2 out]
              }
              frame #1 {
                n221 = local read "Current X (um)"() -> (w476:ext)
                n222 = local read "Current Y (um)"() -> (w475:ext)
                n223 = call "updateFieldnumber - subvi.vi"("Field Size"=w474, "CurY"=w475, "CurX"=w476) -> ("Field Number"=w473:u32)  [unwired: 8 in]
                n224 = local write "Field Number"(w473) -> ()
                n225 = call "field raster.vi"("field size"=w474, "field number"=w473) -> ("Plot1"=w478:cluster{dbl[], dbl[]}, "Plot2"=w477:cluster{dbl[], dbl[]}, "x mark"=w480:dbl[], "y mark"=w481:dbl[])  [unwired: 12 in, 2 out]
                n226 = property on="Current (X,Y)" class="XYGraph (strict)"("XScale.MarkerVals[]"=w480, "YScale.MarkerVals[]"=w481) -> (error out=w479:errorcluster)  [unwired: 2 in, 1 out]
                n227 = call <vilib>:"Simple Error Handler.vi"("error in (no error)"=w479) -> ()  [unwired: 4 in, 5 out]
              }
            }
            n228 = local read "Current Z (um)"() -> (w468:ext)
          }
          event "Field Number": Value Change {
            n229 = event-data() -> ()  [unwired: 7 out]
            n230 = local write "Current Z 2"(0.0) -> ()
            n231 = local read "Field Size"() -> (w494:enum16{"0", "1", "4", "9", "16"})
            n232 = global read "stage-controller-globals.vi" "Previous\nsmall Z increment"() -> (w484:T3)
            n233 = local read "Current Z (um)"() -> (w485:ext)
            n234 = Square(x=w494) -> (x^2=w493:u16)
            n235 = Subtract(x=w485, y=w484) -> (x-y=w483:ext)
            n236 = call "field raster.vi"("field size"=w493, "field number"="Field Number") -> ("Plot1"=w490:cluster{dbl[], dbl[]}, "Plot2"=w489:cluster{dbl[], dbl[]}, "current Y"=w487:dbl, "current X"=w488:dbl)  [unwired: 12 in, 2 out]
          }
        }
        n237 = global read "stage-controller-globals.vi" "Ymax"() -> (w33:dbl)
        n238 = global read "stage-controller-globals.vi" "Xmax"() -> (w34:dbl)
        n239 = global read "stage-controller-globals.vi" "Zmax"() -> (w35:dbl)
        n240 = In Range and Coerce(upper limit=w33, x=w58, lower limit=w59) -> (coerced(x)=w32:ext, In Range?=w54:bool)
        "Current Y (um)" <- w32
        n241 = In Range and Coerce(upper limit=w34, x=w57, lower limit=w59) -> (coerced(x)=w31:ext, In Range?=w52:bool)
        "Current X (um)" <- w31
        n242 = In Range and Coerce(upper limit=w35, x=w56, lower limit=w59) -> (coerced(x)=w30:ext, In Range?=w50:bool)
        "Current Z (um)" <- w30
        n243 = call "Nano-drive-usb-SubVI.vi"("Set this axis?"=w47, "Z (um)"=w30, "Y (um)"=w31, "Numeric"=w46, "X (um)"=w32) -> ()  [unwired: 6 in]
        n244 = local write "Current Z"(w30) -> ()
        n245 = Not(x=w54) -> (.not. x?=→"At limit":bool)
        n246 = Not(x=w52) -> (.not. x?=→"At limit 2":bool)
        n247 = Not(x=w50) -> (.not. x?=→"At limit 3":bool)
        n248 = Initialize Array(w31, 1) -> (w41:ext[])
        n249 = Initialize Array(w32, 1) -> (w40:ext[])
        n250 = global write "stage-controller-globals.vi" "Current Z"(w30) -> ()
        n251 = Bundle(w41, w40) -> (w39:cluster{ext[], ext[]})  [unwired: 1 out]
        n252 = global write "stage-controller-globals.vi" "Current X"(w31) -> ()
        n253 = global write "stage-controller-globals.vi" "Current Y"(w32) -> ()
        n254 = Build Array(w39, w38, w37) -> (→"Current (X,Y)":cluster{ext[], ext[]}[])
      }
      n255 = property on="Current Z 2" class="Slide (strict)"(error in=w15, "Scale.Maximum"=1.0 ("Scale.Range:Maximum"), "Scale.Minimum"=-1.0 ("Scale.Range:Minimum"), "Scale.UniformMarker"=TRUE, "Scale.MinorInc"=0.1 ("Scale.Range:Minor Increment"), "Scale.Increment"=0.2 ("Scale.Range:Increment")) -> (error out=w14:errorcluster)  [unwired: 1 in, 1 out]
      n256 = call <vilib>:"Simple Error Handler.vi"("error in (no error)"=w14) -> ()  [unwired: 4 in, 5 out]
    }
    frame #2 {
      n257 = call "MCL Release Handle.vi"("handle"=w496) -> ()  [unwired: 10 in, 1 out]
      n258 = global write "stage-controller-globals.vi" "stage external trigger"(refnum<k0> refnum) -> ()
      n259 = Unregister For Events(event registration refnum=w498) -> (error out=w499:errorcluster)  [unwired: 1 in]
      n260 = Destroy User Event(user event=w497, error in=w499) -> ()  [unwired: 1 out]
    }
  }
